vi "Revision Query.vi"(8 "error in (no error)":errorcluster, 11 "VISA resource name":refnum<visa-resource-name>) -> (0 "error out":errorcluster, 1 "Instrument Firmware Revision":string, 2 "Instrument Driver Revision":string, 3 "VISA resource name out":refnum<visa-resource-name>)   [LabVIEW 2020, in "TDK-Lambda Z.lvlib"]
doc: "Queries the current instrument firmware revision and instrument driver revision.\n\nRefer to the Readme file for detailed driver information including modification history."
uses:
  TDK-Lambda Z.lvlib
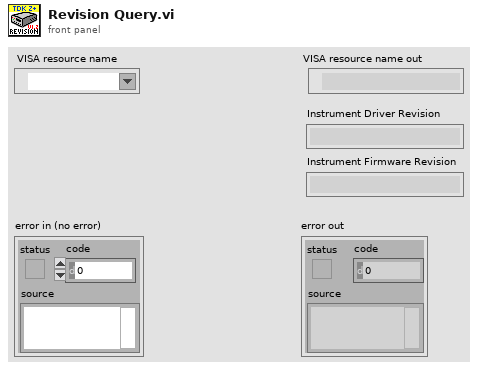
[diagram p1: front panel]
types:
  T1 = enum32{"invalid app kind", "Development System", "Run Time System", "Student Edition", "Embedded LabVIEW", "Evaluation", "Custom"}
  T2 = cluster{"Major":u16, "Minor":u16, "Fix":u16, "Build":u16}
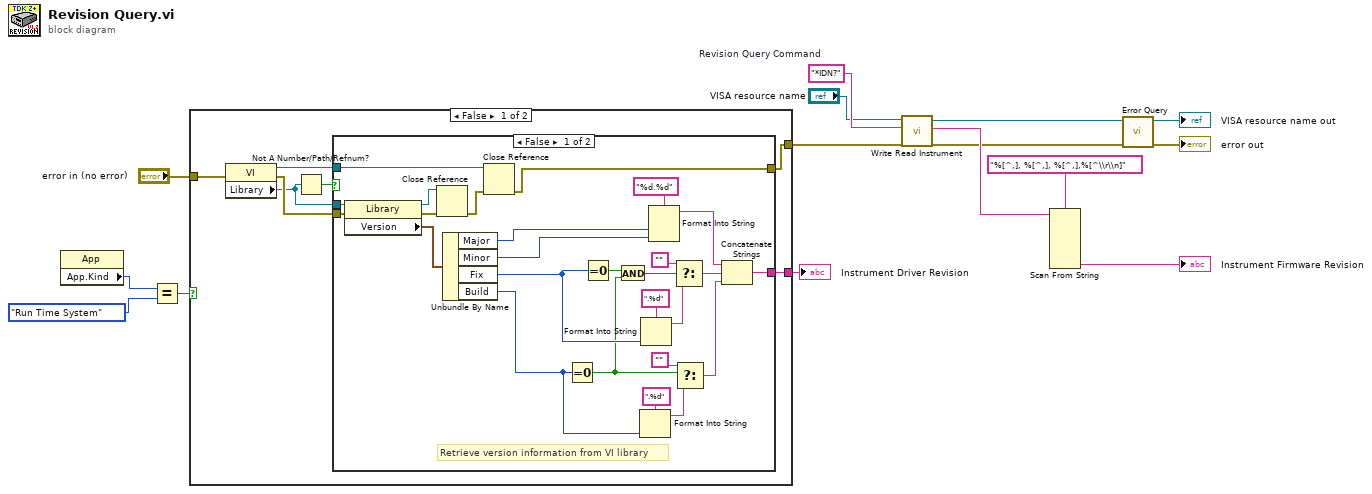
[diagram p0: block diagram]
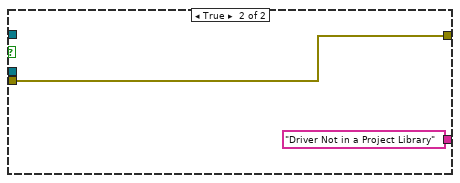
[diagram p2: hidden frame]
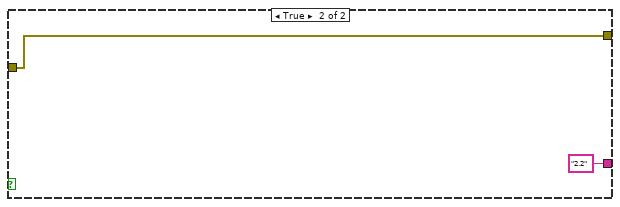
[diagram p3: hidden frame]
diagram:
  w6 = "*IDN?"  # Revision Query Command
  n1 = property class="App"() -> ("App.Kind"=w8:T1)  [unwired: 2 in, 2 out]
  n2 = Equal?(x=w8, y=T1."Run Time System" ("Application:Kind")) -> (x = y?=w9:bool)
  n3 = case shown="False" w9 {
    tunnel: [w18 "2.2"] -> w11
    tunnel: "error in (no error)" -> [w17 w51]
    tunnel: [w16 w51] -> w4
    frame False {
      n4 = property class="VI"(error in=w17) -> (reference out=w22:refnum<vi>, error out=w21:errorcluster, "Library"=w20:refnum<vi>)  [unwired: 1 in]
      n5 = Not A Number/Path/Refnum?(number/path/refnum=w20) -> (NaN/Path/Refnum?=w19:bool)
      n6 = case shown="False" w19 {
        tunnel: w22 -> [w45 _]
        tunnel: w21 -> [w30 w50]
        tunnel: [w25 w50] -> w16
        tunnel: [w24 "Driver Not in a Project Library"] -> w18
        tunnel: w20 -> [w23 _]
        frame False {
          # "Retrieve version information from VI library"
          n7 = property class="Library"(reference=w23, error in=w30) -> (reference out=w47:refnum<vi>, error out=w48:errorcluster, "Version"=w44:T2)
          n8 = Close Reference(reference=w47, error in (no error)=w48) -> (error out=w46:errorcluster)
          n9 = Unbundle By Name(w44) -> ("Major"=w33:u16, "Minor"=w32:u16, "Fix"=w29:u16, "Build"=w31:u16)
          n10 = Close Reference(reference=w45, error in (no error)=w46) -> (error out=w25:errorcluster)
          n11 = Equal To 0?(x=w31) -> (x = 0?=w27:bool)
          n12 = Equal To 0?(x=w29) -> (x = 0?=w28:bool)
          n13 = And(x=w28, y=w27) -> (x .and. y?=w26:bool)
          n14 = Format Into String(format string=".%d", w31) -> (resulting string=w37:string)  [unwired: 2 in, 1 out]
          n15 = Format Into String(format string=".%d", w29) -> (resulting string=w41:string)  [unwired: 2 in, 1 out]
          n16 = Format Into String(format string="%d.%d", w33, w32) -> (resulting string=w39:string)  [unwired: 2 in, 1 out]
          n17 = Select(t="", s=w26, f=w41) -> (s? t:f=w38:string)
          n18 = Select(t="", s=w27, f=w37) -> (s? t:f=w34:string)
          n19 = Concatenate Strings(w39, w38, w34) -> (w24:string)
        }
        frame True {
        }
      }
    }
    frame True {
    }
  }
  "Instrument Driver Revision" <- w11
  n20 = call "Write Read Instrument.vi"("error in (no error)"=w4, "SCPI  Write Command/Query"=w6, "VISA resource name"="VISA resource name") -> ("error out"=w1:errorcluster, "Response"=w2:string, "VISA resource name out"=w3:refnum<visa-resource-name>)  [unwired: 6 in]
  n21 = Scan From String(format string="%[^,], %[^,], %[^,],%[^\\r\\n]", input string=w2) -> (output 4=→"Instrument Firmware Revision":string)  [unwired: 9 in, 3 out]
  n22 = call "Error Query.vi"("error in (no error)"=w1, "VISA resource name"=w3) -> ("error out"=→"error out":errorcluster, "VISA resource name out"=→"VISA resource name out":refnum<visa-resource-name>)  [unwired: 6 in, 2 out]
